vi "Wrap in Quotes.vi"(11 "String":string) -> (3 "String with Quotes":string)   [LabVIEW 2015, in "NI_Azure_JSON Parsing.lvlib"]
uses:
  NI_Azure_JSON Parsing.lvlib
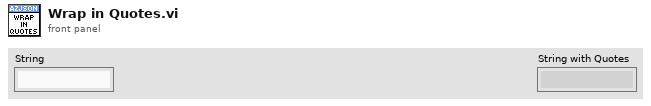
[diagram p1: front panel]
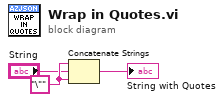
[diagram p0: block diagram]
diagram:
  w2 = "\""
  n1 = Concatenate Strings(w2, "String", w2) -> (→"String with Quotes":string)
